vi "VFH-r140_probe_values.vi"(9 "L":dbl=0.05 format="%#_13p", 10 "R2 B":dbl=0.00175 format="%#_13p", 11 "R1 A":dbl=0.000465 format="%#_13p") -> (2 "result":dbl)   [LabVIEW 2020, in "VFH-VNA_File_Handler.lvlib"]
uses:
  VFH-VNA_File_Handler.lvlib
panel:
  # "0.00175"
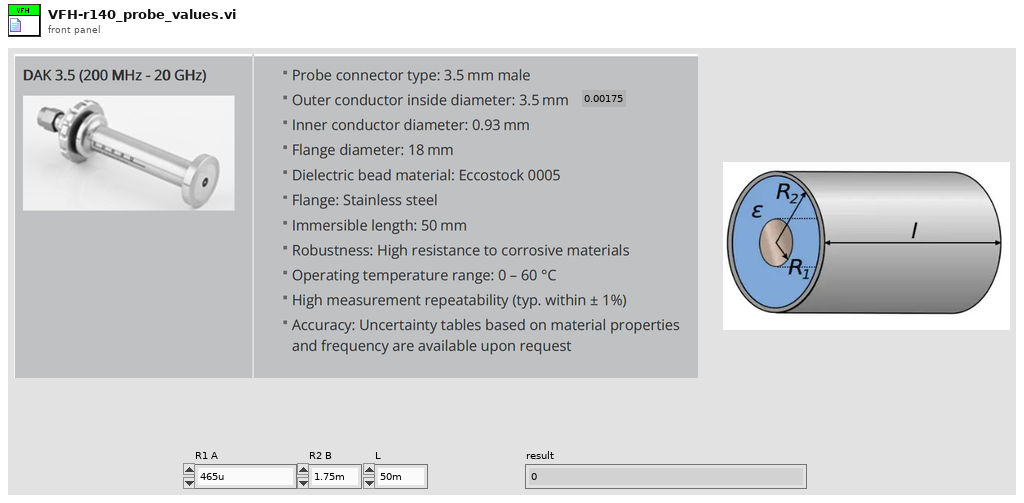
[diagram p1: front panel]
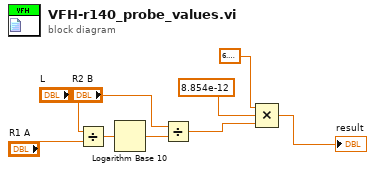
[diagram p0: block diagram]
diagram:
  n1 = Divide(x="R2 B", y="R1 A") -> (x/y=w5:dbl)
  n2 = Logarithm Base 10(1:w5) -> (0:w6:dbl)
  n3 = Divide(x="L", y=w6) -> (x/y=w2:dbl)
  n4 = Compound Arithmetic op=MULTIPLY(6.283185307179586, 8.854e-12, w2) -> (→"result":dbl)
